vi "Check file size.vi"(8 "error in (no error)":errorcluster, 10 "min size (KB)":i64, 11 "DAQOrcaFlash in":refnum<class "DAQOrcaFlash.lvclass">) -> (0 "error out":errorcluster, 2 "too small?":bool, 3 "DAQOrcaFlash out":refnum<class "DAQOrcaFlash.lvclass">)   [LabVIEW 2012, in "DAQOrcaFlash.lvclass"]
uses:
  DAQOrcaFlash.lvclass
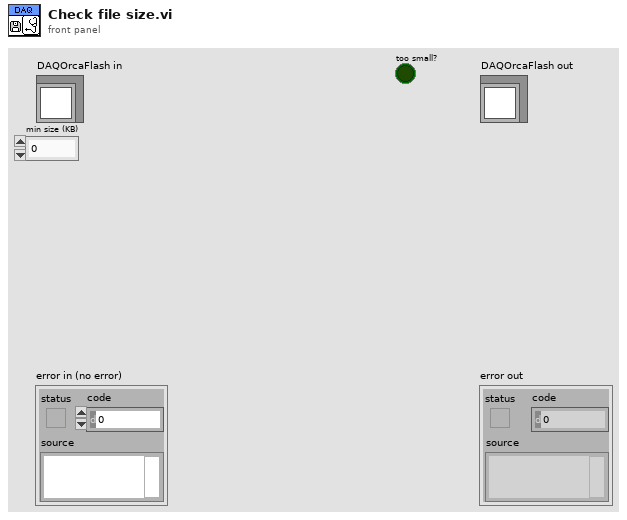
[diagram p1: front panel]
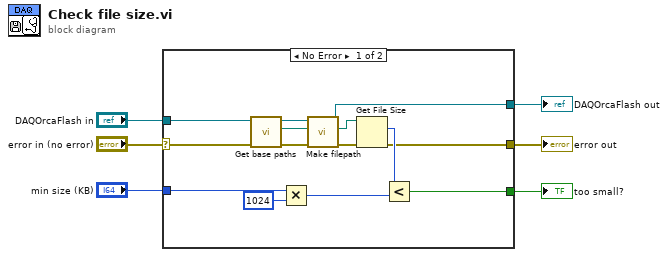
[diagram p0: block diagram]
diagram:
  n1 = case shown="No Error" "error in (no error)" {
    selector: "error in (no error)" -> [w16 w22]
    tunnel: [w7 w22] -> w5
    tunnel: [w8 w21] -> w3
    tunnel: "DAQOrcaFlash in" -> [w17 w21]
    tunnel: "min size (KB)" -> [w12 _]
    tunnel: [w9 _] -> w1
    frame No Error {
      n2 = call-dynamic "Get base paths.vi"("error in (no error)"=w16, "DAQOrcaFlash in"=w17) -> ("error out"=w20:errorcluster, "filepath"=w18:path, "DAQOrcaFlash out"=w19:refnum<class "DAQOrcaFlash.lvclass">)  [unwired: 6 in, 1 out]
      n3 = Multiply(x=w12, y=i64 1024 ("size (in bytes)")) -> (x*y=w10:i64)
      n4 = call "Make filepath.vi"("error in (no error)"=w20, "base path"=w18, "DAQOrcaFlash in"=w19) -> ("error out"=w15:errorcluster, "filepath out"=w14:path, "DAQOrcaFlash out"=w8:refnum<class "DAQOrcaFlash.lvclass">)  [unwired: 6 in]
      n5 = Get File Size(file=w14, error in=w15) -> (size (in bytes)=w11:i64, 0:w7:errorcluster)  [unwired: 1 out]
      n6 = Less?(x=w11, y=w10) -> (x < y?=w9:bool)
    }
    frame Error {
    }
  }
  "error out" <- w5
  "DAQOrcaFlash out" <- w3
  "too small?" <- w1
